vi "Change List Font Size.vi"(8 "error in":errorcluster, 10 "Char":i16, 11 "MulticolumnListbox in":refnum<vi>) -> (0 "error out":errorcluster)   [LabVIEW 2016]
uses:
  <vilib>/Utility/miscctls.llb/LVRowAndColumnTypeDef.ctl
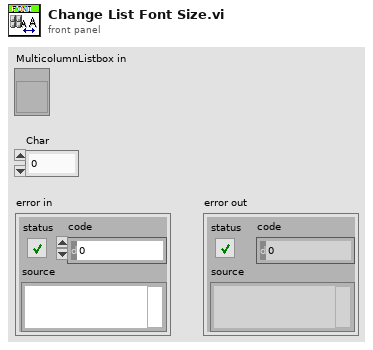
[diagram p1: front panel]
types:
  T1 = typedef "LVRowAndColumnTypeDef.ctl" = cluster{"Row":i32, "Column":i32}
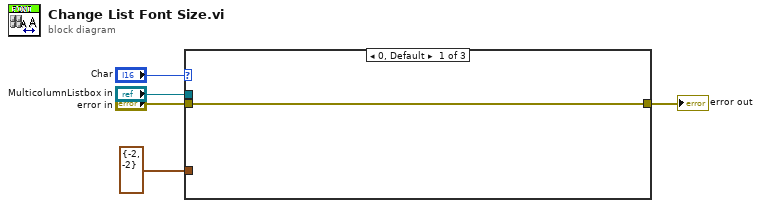
[diagram p0: block diagram]
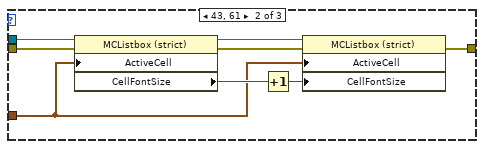
[diagram p2: hidden frame]
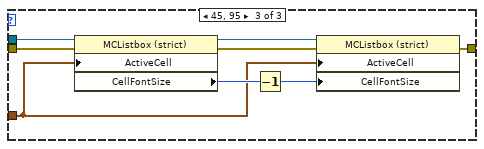
[diagram p3: hidden frame]
diagram:
  n1 = case shown="0, Default" "Char" {
    tunnel: "MulticolumnListbox in" -> [_ w14 w19]
    tunnel: T1 {"Row"=-2, "Column"=-2} ("Active Cell:Active Cell") -> [_ w10 w18]
    tunnel: "error in" -> [w6 w7 w17]
    tunnel: [w6 w8 w15] -> w1
    frame 0, Default {
    }
    frame 43, 61 {
      n2 = property class="MCListbox (strict)"(reference=w14, error in=w7, "ActiveCell"=w10) -> (reference out=w13:refnum<vi>, error out=w9:errorcluster, "CellFontSize"=w12:u32)
      n3 = Increment(x=w12) -> (x+1=w11:u32)
      n4 = property class="MCListbox (strict)"(reference=w13, error in=w9, "ActiveCell"=w10, "CellFontSize"=w11) -> (error out=w8:errorcluster)  [unwired: 1 out]
    }
    frame 45, 95 {
      n5 = property class="MCListbox (strict)"(reference=w19, error in=w17, "ActiveCell"=w18) -> (reference out=w22:refnum<vi>, error out=w16:errorcluster, "CellFontSize"=w21:u32)
      n6 = Decrement(x=w21) -> (x-1=w20:u32)
      n7 = property class="MCListbox (strict)"(reference=w22, error in=w16, "ActiveCell"=w18, "CellFontSize"=w20) -> (error out=w15:errorcluster)  [unwired: 1 out]
    }
  }
  "error out" <- w1
